vi "Var2Class.vi"(7 "ClassType":refnum<class>, 10 "error in":errorcluster, 11 "ExpectedType":variant) -> (2 "error out":errorcluster, 3 "object out":refnum<class>)   [LabVIEW 2020, in "ORM.lvlib" / "TypeMap.lvclass"]
uses:
  TypeMap.lvclass
  TypeMap.lvclass/TypeMap.ctl
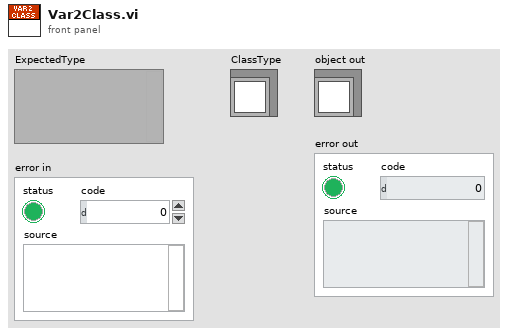
[diagram p1: front panel]
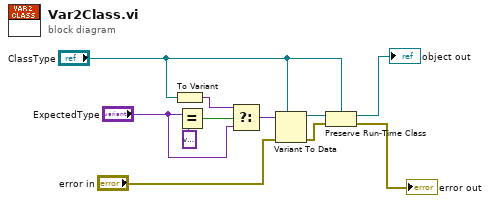
[diagram p0: block diagram]
diagram:
  n1 = To Variant(anything="ClassType") -> (Variant=w8:variant)
  n2 = Equal?(x="ExpectedType", y=variant) -> (x = y?=w10:bool)
  n3 = Select(t=w8, s=w10, f="ExpectedType") -> (s? t:f=w7:variant)
  n4 = Variant To Data(error in="error in", type="ClassType", Variant=w7) -> (data=w6:refnum<class>, error out=w5:errorcluster)
  n5 = Preserve Run-Time Class(object in=w6, error in=w5, 2:"ClassType") -> (object out=→"object out":refnum<class>, error out=→"error out":errorcluster)
